vi "Tx.vi"(6 "TermChar (\\r\\n)":string="\r\n", 8 "error in":errorcluster, 10 "Command":string, 11 "VISA in":refnum<visa-resource-name>) -> (0 "error out":errorcluster, 3 "VISA out":refnum<visa-resource-name>)   [LabVIEW 2016, in "Serial_G.lvlib"]
doc: "Write to VISA"
uses:
  Serial_G.lvlib
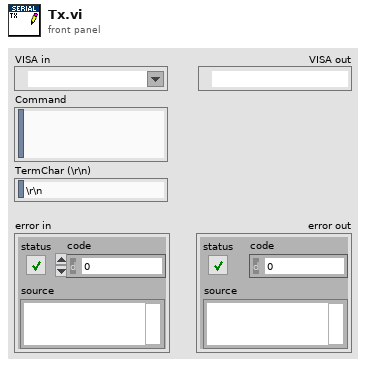
[diagram p1: front panel]
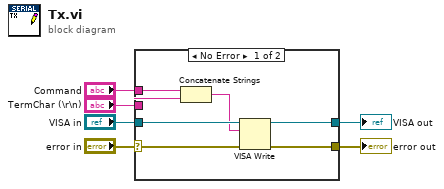
[diagram p0: block diagram]
diagram:
  n1 = case shown="No Error" "error in" {
    selector: "error in" -> [w13 w15]
    tunnel: [w12 w15] -> w6
    tunnel: "VISA in" -> [w11 w14]
    tunnel: "Command" -> [w10 _]
    tunnel: [w9 w14] -> w2
    tunnel: "TermChar (\\r\\n)" -> [w7 _]
    frame No Error {
      n2 = Concatenate Strings(w10, w7) -> (w8:string)
      n3 = VISA Write(VISA resource name=w11, write buffer=w8, error in (no error)=w13) -> (VISA resource name out=w9:refnum<visa-resource-name>, error out=w12:errorcluster)  [unwired: 1 out]
    }
    frame Error {
    }
  }
  "error out" <- w6
  "VISA out" <- w2
